vi "RELEASE - 1.0 - Motor Limitter - David G.vi"(5 "refnum name":string="Encoder Lift", 8 "Backward Speed":dbl=0.7 format="%#_13g", 9 "Forward Speed":dbl=0.7 format="%#_13g", 10 "Backward Limit":dbl=0.7 format="%#_13g", 11 "Forward Limit":dbl=0.7 format="%#_13g") -> (1 "Backward Value":dbl=20.0 format="%#_13g", 2 "Forward Value":dbl=20.0 format="%#_13g", 4 "Encoder Value":dbl=20.0 format="%#_13g")   [LabVIEW 2018]
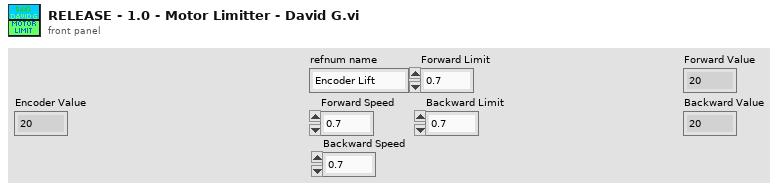
[diagram p1: front panel]
types:
  T1 = typedef "WPI_EncoderDevRef.ctl" = cluster{"DevStatus":errorcluster, "EncoderIndex":T2, "CounterIndex":T3, "DistancePerCount":dbl, "Decoding Type":T4}
  T2 = typedef "FPGA_EncoderIdx.ctl" = enum8{"Enc 0", "Enc 1", "Enc 2", "Enc 3", "Enc 4", "Enc 5", "Enc 6", "Enc 7", "Invalid"}
  T3 = typedef "FPGA_CounterCtrSystemIndex.ctl" = enum8{"Ctr 0", "Ctr 1", "Ctr 2", "Ctr 3", "Ctr 4", "Ctr 5", "Ctr 6", "Ctr 7", "Invalid"}
  T4 = typedef "WPI_EncoderType.ctl" = enum16{"1x", "2x", "4x"}
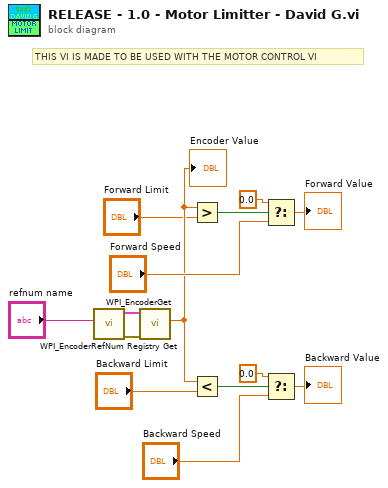
[diagram p0: block diagram]
diagram:
  # "THIS VI IS MADE TO BE USED WITH THE MOTOR CONTROL VI"
  n1 = call <vilib>:"WPI_EncoderRefNum Registry Get.vi"("refnum name"="refnum name") -> ("error out"=w14:errorcluster, "EncoderDevRef"=w13:T1)  [unwired: 9 in]
  n2 = call <vilib>:"WPI_EncoderGet.vi"("error in (no error)"=w14, "EncoderDevRef"=w13) -> ("Distance"=w6:dbl)  [unwired: 4 in, 5 out]
  "Encoder Value" <- w6
  n3 = Greater?(x=w6, y="Forward Limit") -> (0:w11:bool)
  n4 = Less?(x=w6, y="Backward Limit") -> (x < y?=w10:bool)
  n5 = Select(t=0.0 ("f"), s=w11, f="Forward Speed") -> (s? t:f=→"Forward Value":dbl)
  n6 = Select(t=0.0 ("f"), s=w10, f="Backward Speed") -> (s? t:f=→"Backward Value":dbl)
